vi "Read Channel Array.vi"(8 "error in":errorcluster, 10 "channels":refnum<class "Channel.lvclass">[](array[class]), 11 "thermocouple mode in":refnum<class "Thermocouple Mode.lvclass">) -> (0 "error out":errorcluster, 2 "channel settings":T1[](array[typedef]), 3 "thermocouple mode out":refnum<class "Thermocouple Mode.lvclass">)   [LabVIEW 2020, in "Scan Engine Scripting.lvlib" / "Thermocouple Mode.lvclass"]
uses:
  Thermocouple Mode.lvclass
  Channel Classes/Channel/Channel.lvclass
  Controls/thermocouple channel settings.ctl
  Channel Classes/Thermocouple Channel/Thermocouple Type.ctl
  Channel Classes/Thermocouple Channel/Measurement Units.ctl
  Channel Classes/Thermocouple Channel/Thermocouple Channel.lvclass
  Scan Engine Scripting.lvlib
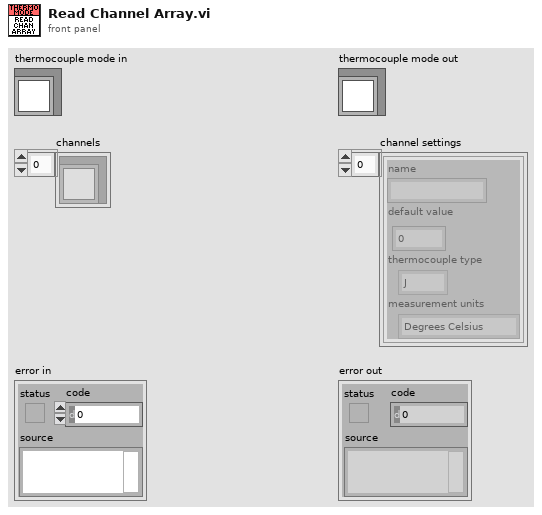
[diagram p1: front panel]
types:
  T1 = typedef "Scan Engine Scripting.lvlib/thermocouple channel settings.ctl" = cluster{"name":string, "default value":dbl, "thermocouple type":T2, "measurement units":T3}
  T2 = typedef "Scan Engine Scripting.lvlib/Thermocouple Channel.lvclass/Thermocouple Type.ctl" = enum16{"J", "K", "T", "E", "R", "S", "N", "B"}
  T3 = typedef "Scan Engine Scripting.lvlib/Thermocouple Channel.lvclass/Measurement Units.ctl" = enum16{"Raw Volts", "Degrees Kelvin", "Degrees Celsius", "Degrees Fahrenheit", "Degrees Rankine"}
  T4 = typedef "Scan Engine Scripting.lvlib/Thermocouple Channel.lvclass/Thermocouple Channel Settings.ctl" = cluster{"thermocouple type":T2, "measurement units":T3}
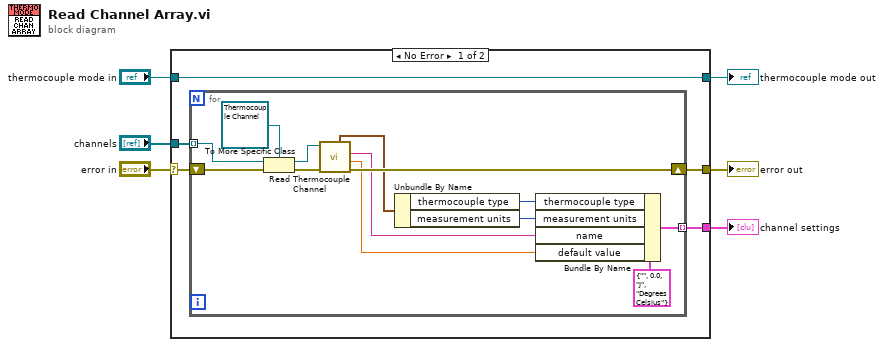
[diagram p0: block diagram]
diagram:
  n1 = case shown="No Error" "error in" {
    selector: "error in" -> [w9 w26]
    tunnel: [w8 w26] -> w5
    tunnel: [w11 w25] -> w3
    tunnel: "thermocouple mode in" -> [w11 w25]
    tunnel: "channels" -> [w10 _]
    tunnel: [w7 _] -> w1
    frame No Error {
      n2 = for {
        tunnel: w10 -> [w21] mode=indexing
        tunnel: [w23] -> w7 mode=indexing
        shift-right: [w20] -> w8
        shift-left: w9 -> [w22]
        n3 = To More Specific Class(target class=refnum<class "Thermocouple Channel.lvclass"> refnum ("Scan Engine Scripting.lvlib:Thermocouple Channel.lvclass"), reference=w21, error in=w22) -> (specific class reference=w15:refnum<class "Thermocouple Channel.lvclass">, error out=w19:errorcluster)
        n4 = call "Read Thermocouple Channel.vi"("error in"=w19, "thermocouple channel in"=w15) -> ("error out"=w20:errorcluster, "default value"=w17:dbl, "name"=w18:string, "thermocouple channel settings"=w14:T4)  [unwired: 4 in, 2 out]
        n5 = Unbundle By Name(w14) -> ("thermocouple type"=w13:T2, "measurement units"=w12:T3)
        n6 = Bundle By Name(cluster=T1 {"name"="", "default value"=0.0, "thermocouple type"=enum."J", "measurement units"=enum."Degrees Celsius"} ("channel settings"), "thermocouple type"=w13, "measurement units"=w12, "name"=w18, "default value"=w17) -> (w23:T1)
      }
    }
    frame Error {
    }
  }
  "error out" <- w5
  "thermocouple mode out" <- w3
  "channel settings" <- w1
